vi "RS_SMBV100A_ADD_ACCELERATION.vi"(2 "COUNT IN":dbl format="%#_13g", 3 "Scenario Name Previous":string="ACCELERATION", 4 "Scenario Name New in":string="LINE", 5 "RESOLUTION":dbl=0.1 format="%#_13g") -> (0 "COUNT OUT":dbl, 1 "Scenario Name New out":string)   [LabVIEW 2018]
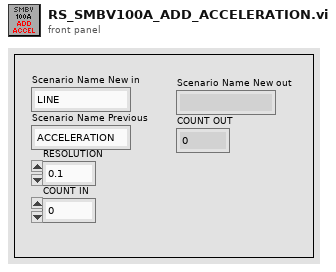
[diagram p1: front panel]
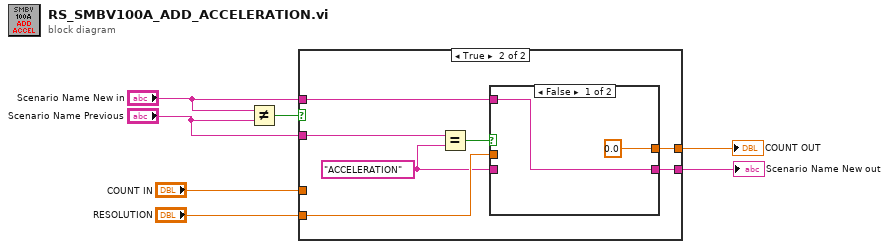
[diagram p0: block diagram]
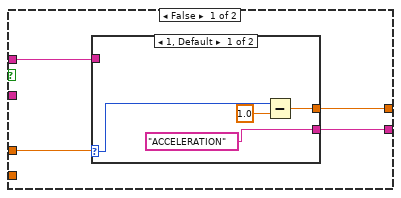
[diagram p2: hidden frame]
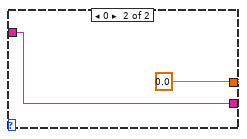
[diagram p3: hidden frame]
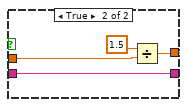
[diagram p4: hidden frame]
diagram:
  n1 = Not Equal?(x="Scenario Name New in", y="Scenario Name Previous") -> (x != y?=w7:bool)
  n2 = case shown="True" w7 {
    tunnel: "Scenario Name Previous" -> [_ w24]
    tunnel: "RESOLUTION" -> [_ w22]
    tunnel: "Scenario Name New in" -> [w10 w20]
    tunnel: [w9 w18] -> w3
    tunnel: "COUNT IN" -> [w11 _]
    tunnel: [w8 w21] -> w1
    frame False {
      n3 = case shown="1, Default" w11 {
        selector: w11 -> [w13 _]
        tunnel: w10 -> [_ w17]
        tunnel: ["ACCELERATION" w17] -> w9
        tunnel: [w12 0.0] -> w8
        frame 1, Default {
          n4 = Subtract(x=w13, y=1.0) -> (x-y=w12:dbl)
        }
        frame 0 {
        }
      }
    }
    frame True {
      w19 = "ACCELERATION"
      n5 = Equal?(x=w24, y=w19) -> (x = y?=w23:bool)
      n6 = case shown="False" w23 {
        tunnel: w22 -> [_ w29]
        tunnel: [0.0 w28] -> w21
        tunnel: w20 -> [w25 _]
        tunnel: [w25 w27] -> w18
        tunnel: w19 -> [_ w27]
        frame False {
        }
        frame True {
          n7 = Divide(x=1.5, y=w29) -> (x/y=w28:dbl)
        }
      }
    }
  }
  "Scenario Name New out" <- w3
  "COUNT OUT" <- w1
